vi "FM Receiver - 副本.vi"() -> ()   [LabVIEW 2013]
doc: "Use this template to build a producer/consumer design pattern. Use this template when you need to execute a process, such as data analysis, when a data source, such as a triggered acquisition, produces data at an uneven rate and you need to execute the process when the data becomes available."
uses:
  <vilib>/Waveform/WDTFileIO.llb/Read Waveform from File.vi
  <vilib>/Analysis/NI_AALPro.lvlib
  <vilib>/Analysis/2dsp.llb/Rational Resample (single channel, DBL).vi
  <vilib>/sound2/lvsound2.llb/Sound Output Write (DBL Single).vi
  <userlib>/FMDemoRTLSDR_DLL/FMDemoRTLSDR_DLL.lvlib
panel:
  in  "Name":cluster{"Decimation":u32, "Interpolation":u32}
  out "error out":errorcluster
  in  "Sound format":T1
  in  "IQ Rate":u32
  out "Waveform":waveform(dbl)(graph)
  out "error out":errorcluster
  in  "file path (dialog if empty)":path
  in  "stop":bool
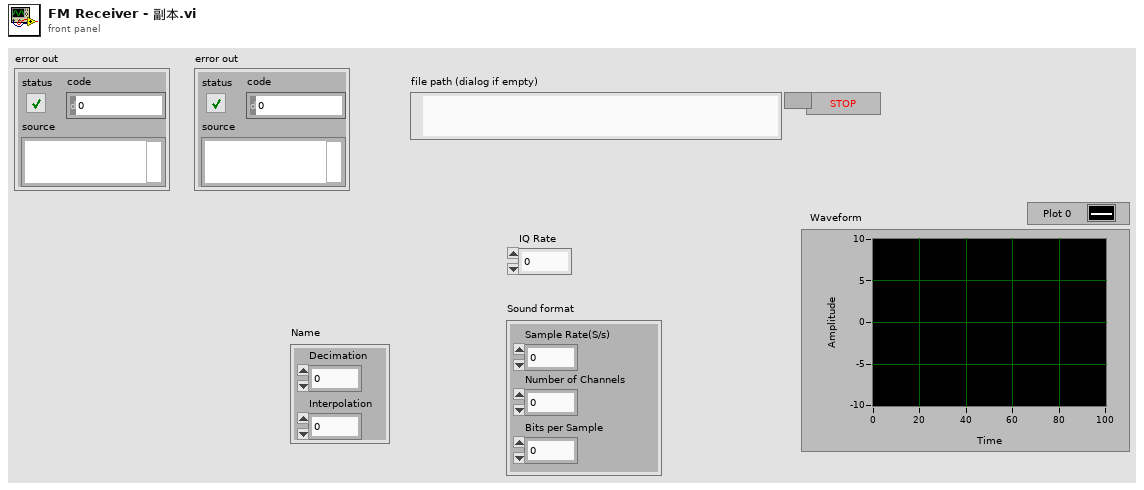
[diagram p1: front panel]
types:
  T1 = cluster{"Sample Rate(S/s)":dbl, "Number of Channels":dbl, "Bits per Sample":dbl}
  T2 = typedef "Sound Output Task ID.ctl" = u32
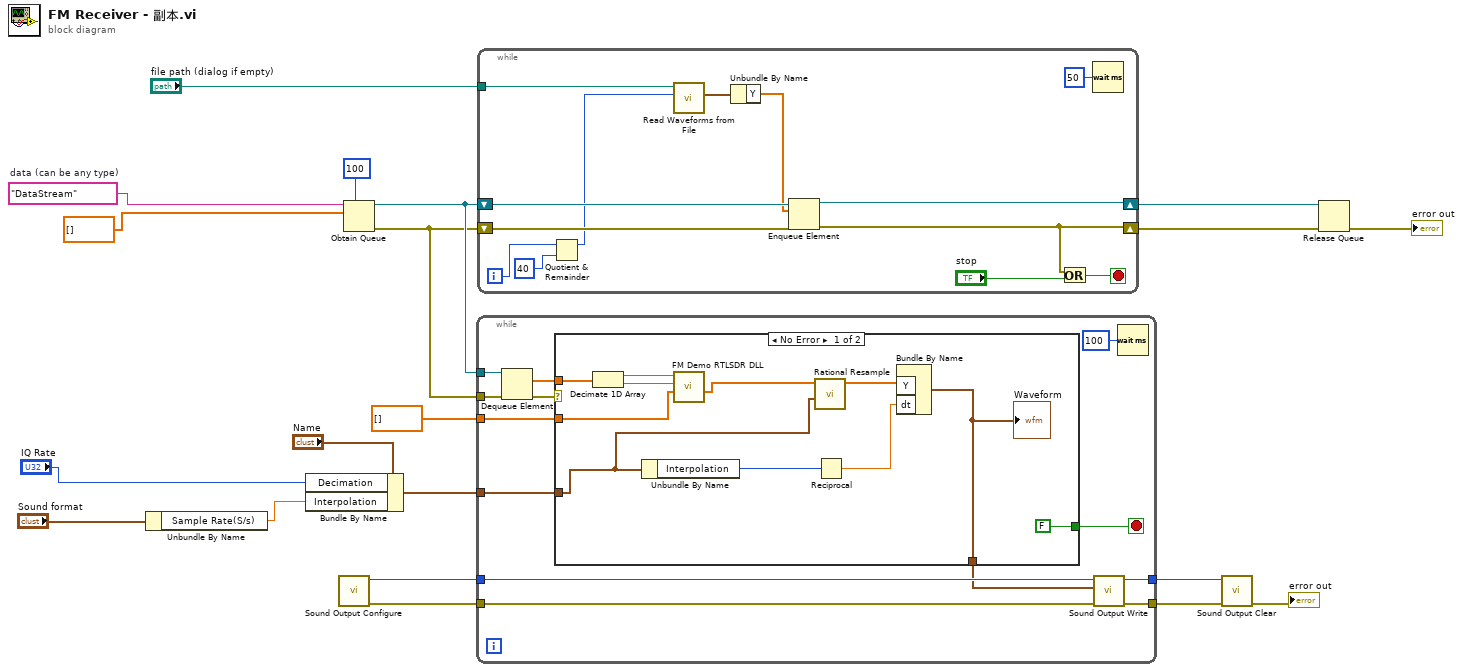
[diagram p0: block diagram]
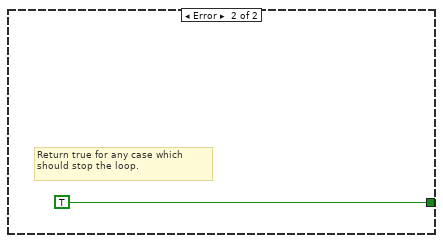
[diagram p2: hidden frame]
diagram:
  w13 = "DataStream"  # data (can be any type)
  n1 = Unbundle By Name("Sound format") -> ("Sample Rate(S/s)"=w5:dbl)
  n2 = Bundle By Name(cluster="Name", "Decimation"="IQ Rate", "Interpolation"=w5) -> (w1:cluster{"Decimation":u32, "Interpolation":u32})
  n3 = call <vilib>:"Sound Output Configure.vi"() -> ("error out"=w9:errorcluster, "task ID"=w7:T2)  [unwired: 10 in]
  n4 = Obtain Queue(max queue size (-1, unlimited)=100, name (unnamed)=w13, element data type=dbl[] []) -> (queue out=w20:refnum<queue>, error out=w14:errorcluster)  [unwired: 2 in, 1 out]
  n5 = while {
    tunnel: w20 -> [w33]
    tunnel: w14 -> [w29]
    tunnel: [w27] -> w11
    tunnel: [w26] -> w10
    tunnel: w9 -> [w25]
    tunnel: w7 -> [w24]
    tunnel: dbl[] [] -> [w22]
    tunnel: w1 -> [w21]
    stop <- w30 stop-if-true
    n6 = Dequeue Element(queue=w33, error in (no error)=w29) -> (element=w31:dbl[], error out=w32:errorcluster)  [unwired: 1 in, 2 out]
    n7 = case shown="No Error" w32 {
      tunnel: w31 -> [w43 _]
      tunnel: [FALSE TRUE] -> w30
      tunnel: [w40 _] -> w23
      tunnel: w22 -> [w37 _]
      tunnel: w21 -> [w35 _]
      frame No Error {
        n8 = Decimate 1D Array(w43) -> (w39:dbl[], w38:dbl[])
        n9 = Unbundle By Name(w35) -> ("Interpolation"=w34:u32)
        n10 = call <userlib>:"FM Demo RTLSDR DLL.vi"("Baseband"=w37, "QSamples"=w38, "ISamples"=w39) -> ("Baseband out"=w36:dbl[])  [unwired: 8 in]
        n11 = call-poly <vilib>:"Rational Resample.vi"("resample factor"=w35, "X"=w36) -> ("Y"=w42:dbl[])  [unwired: 7 in, 2 out]
        n12 = Reciprocal(x=w34) -> (1/x=w41:dbl)
        n13 = Bundle By Name("Y"=w42, "dt"=w41) -> (w40:waveform(dbl))  [unwired: 1 in]
        "Waveform" <- w40
      }
      frame Error {
        # "Return true for any case which should stop the loop."
      }
    }
    n14 = call-poly <vilib>:"Sound Output Write.vi"("error in (no error)"=w25, "data"=w23, "task ID"=w24) -> ("error out"=w26:errorcluster, "task ID out"=w27:T2)  [unwired: 7 in]
    n15 = Wait (ms)(milliseconds to wait=u32 100) -> ()  [unwired: 1 out]
  }
  n16 = while {
    shift-right: [w47] -> w18
    shift-left: w14 -> [w54]
    shift-right: [w55] -> w19
    shift-left: w20 -> [w53]
    tunnel: "file path (dialog if empty)" -> [w57]
    i -> [w52]
    stop <- w48 stop-if-true
    n17 = Quotient & Remainder(x=w52, y=40) -> (x-y*floor(x/y)=w50:i32)  [unwired: 1 out]
    n18 = call-poly <vilib>:"Read Waveforms from File.vi"("offset (records:0)"=w50, "file path (dialog if empty)"=w57) -> ("first waveform in record"=w56:waveform(dbl))  [unwired: 4 in, 3 out]
    n19 = Unbundle By Name(w56) -> ("Y"=w49:dbl[])
    n20 = Enqueue Element(queue=w53, element=w49, error in (no error)=w54) -> (queue out=w55:refnum<queue>, error out=w47:errorcluster)  [unwired: 1 in, 1 out]
    n21 = Or(x=w47, y="stop") -> (x .or. y?=w48:bool)
    n22 = Wait (ms)(milliseconds to wait=u32 50) -> ()  [unwired: 1 out]
  }
  n23 = call <vilib>:"Sound Output Clear.vi"("error in (no error)"=w10, "task ID"=w11) -> ("error out"=→"error out":errorcluster)  [unwired: 9 in]
  n24 = Release Queue(queue=w19, error in (no error)=w18) -> (error out=→"error out":errorcluster)  [unwired: 1 in, 2 out]
